vi "UNLOADING_CHECH_STATUS.vi"(0 "Unloading cyc Data":T1) -> (4 "DOOR NO.":string, 6 "QR Code":string, 8 "Unloading cyc Data OUT":T1)   [LabVIEW 2017]
uses:
  Controls/Feed_Cyc_Data.ctl
  Controls/Unloading_Cyc_Data.ctl
  <vilib>/Utility/file.llb/Read Delimited Spreadsheet (string).vi
  <vilib>/Utility/file.llb/Write Delimited Spreadsheet (string).vi
panel:
  in  "error in":errorcluster
  out "error out":errorcluster
  out "?":T2
  in  "Enum":enum16{"FEED", "LOADED"}(ring)=enum."LOADED"
  in  "Door No":i32
  out "output array":string[][](array[string])
  out "error out":errorcluster
  in  "error in (no error)":errorcluster
  in  "?":T2
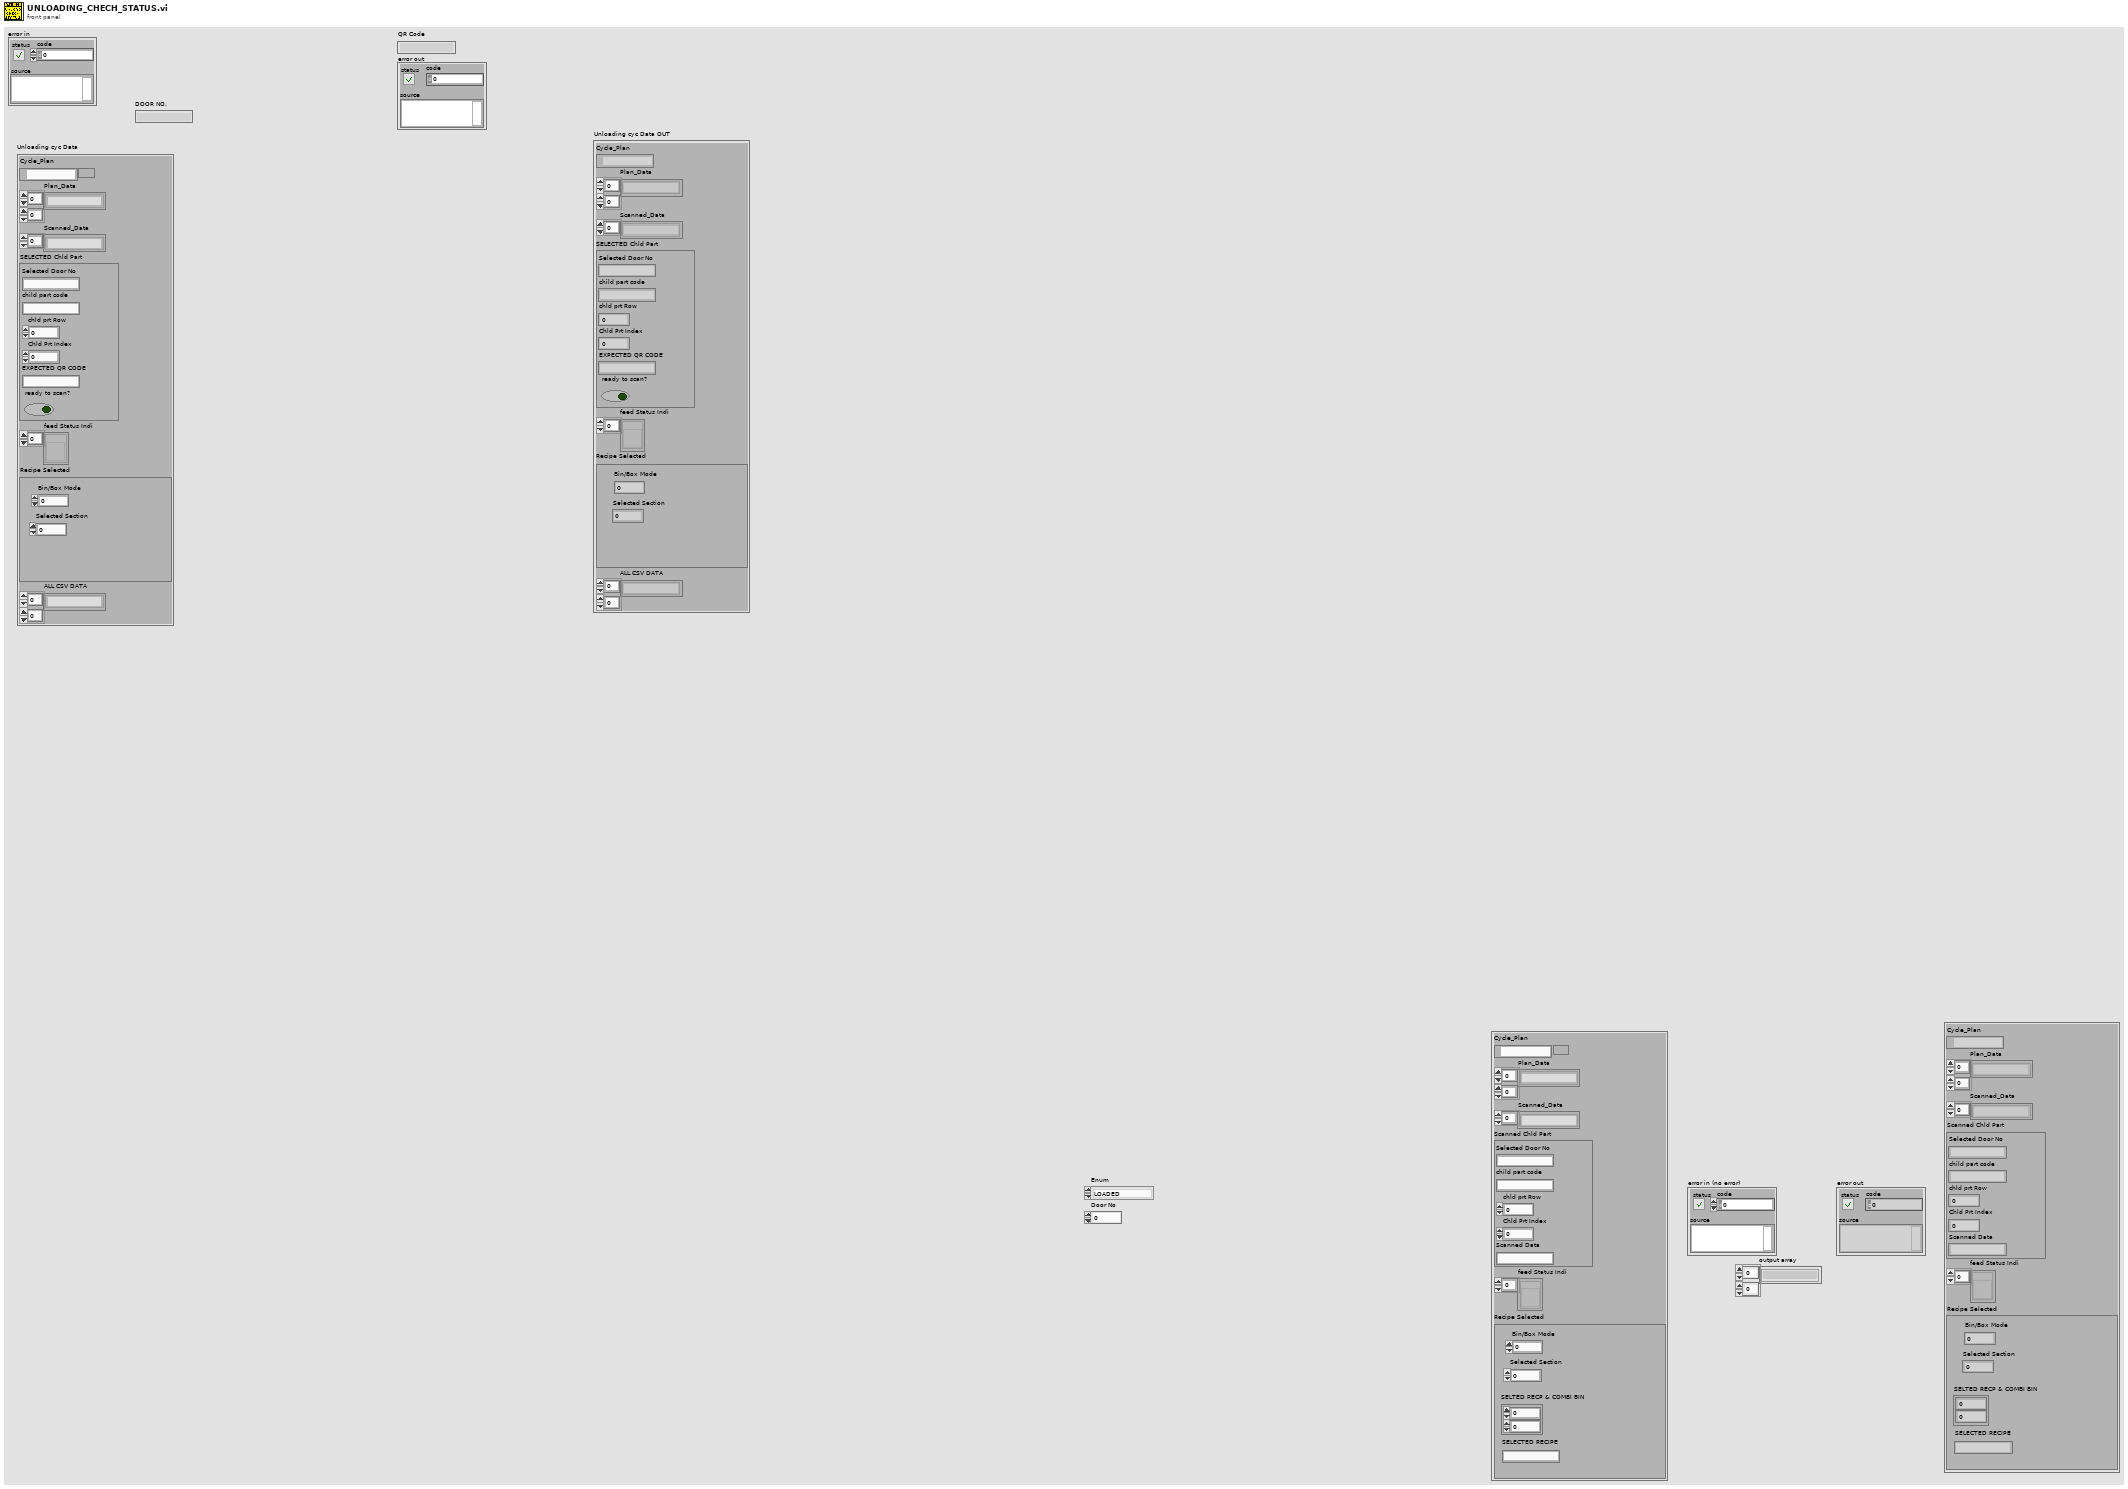
[diagram p1: front panel]
types:
  T1 = typedef "Unloading_Cyc_Data.ctl" = cluster{"Cycle_Plan":path, "Plan_Data":string[][], "Scanned_Data":string[], "SELECTED Chld Part":cluster{"Selected Door No":string, "child part code":string, "chld prt Row":i32, "Chld Prt Index":i32, "EXPECTED QR CODE":string, "ready to scan?":bool}, "feed Status Indi":refnum<vi>[], "Recipe Selected":cluster{"Bin/Box Mode":i32, "Selected Section":i32}, "ALL CSV DATA":string[][]}
  T2 = typedef "Feed_Cyc_Data.ctl" = cluster{"Cycle_Plan":path, "Plan_Data":string[][], "Scanned_Data":string[], "Scanned Chld Part":cluster{"Selected Door No":string, "child part code":string, "chld prt Row":i32, "Chld Prt Index":i32, "Scanned Data":string}, "feed Status Indi":refnum<vi>[], "Recipe Selected":cluster{"Bin/Box Mode":i32, "Selected Section":i32, "SELTED RECP & COMBI BIN":cluster{i32, i32}, "SELECTED RECIPE":string}}
  T3 = cluster{"Selected Door No":string, "child part code":string, "chld prt Row":i32, "Chld Prt Index":i32, "Scanned Data":string}
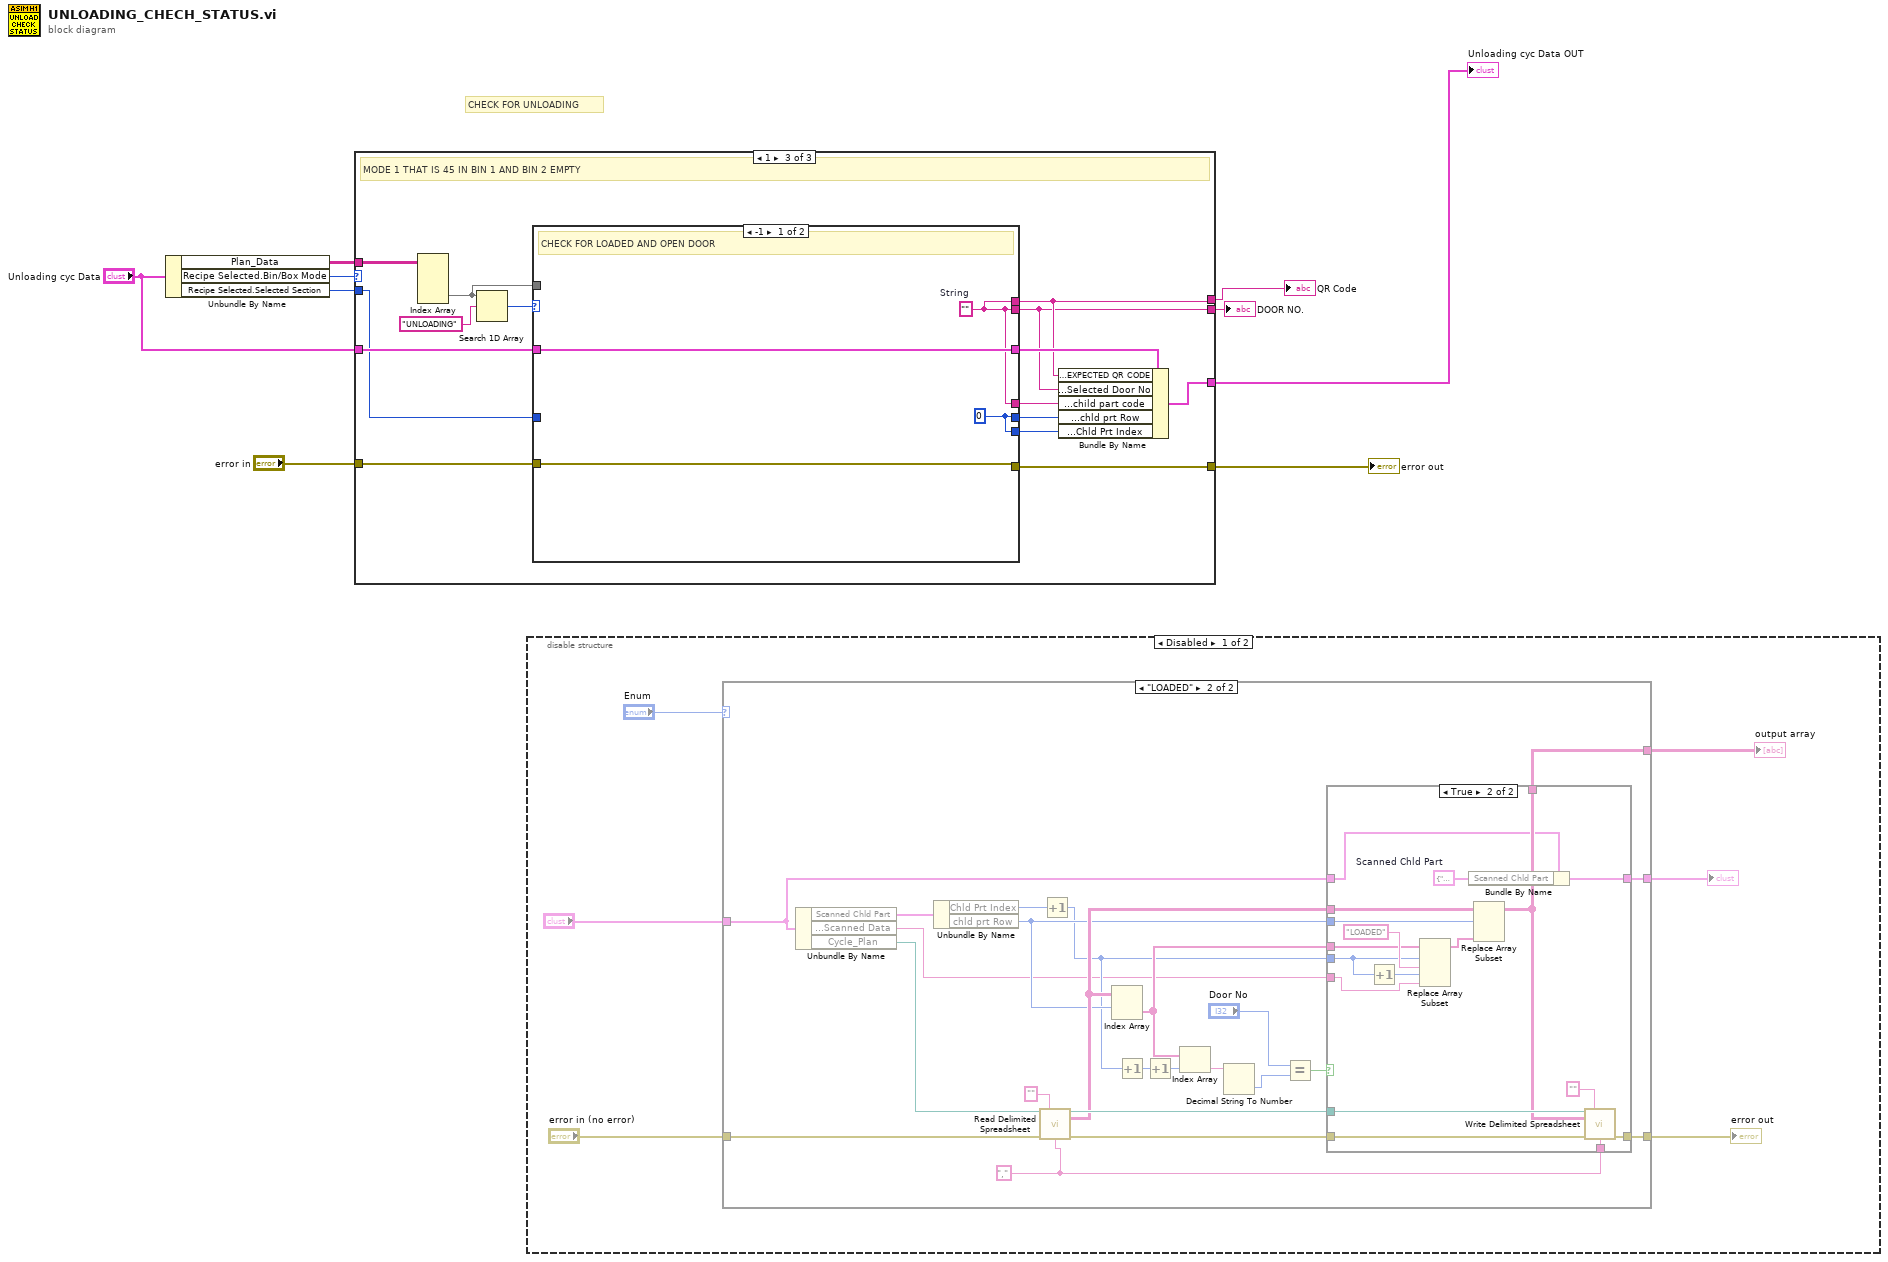
[diagram p0: block diagram]
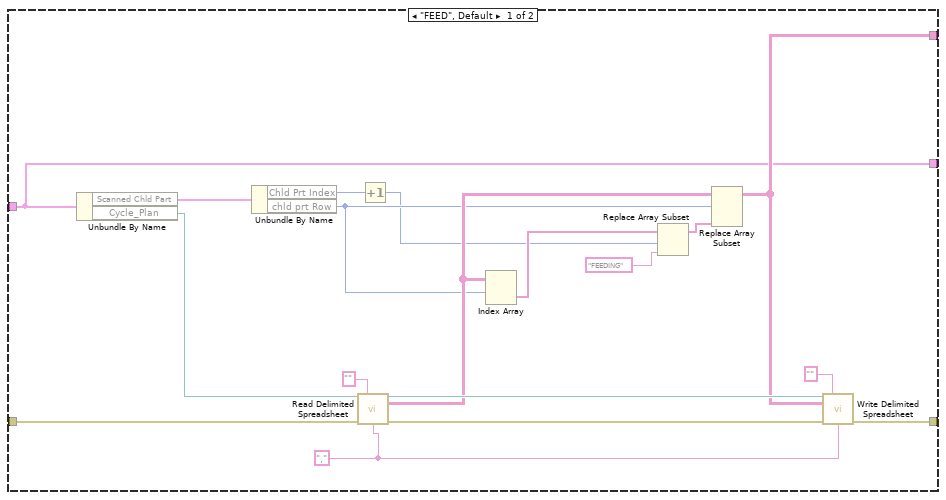
[diagram p2: hidden frame]
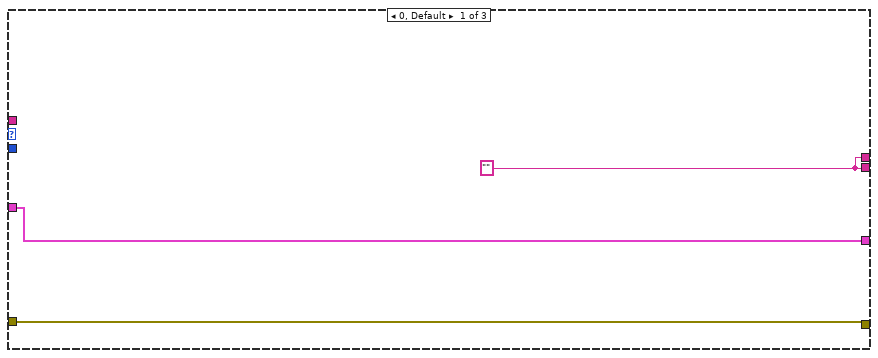
[diagram p5: hidden frame]
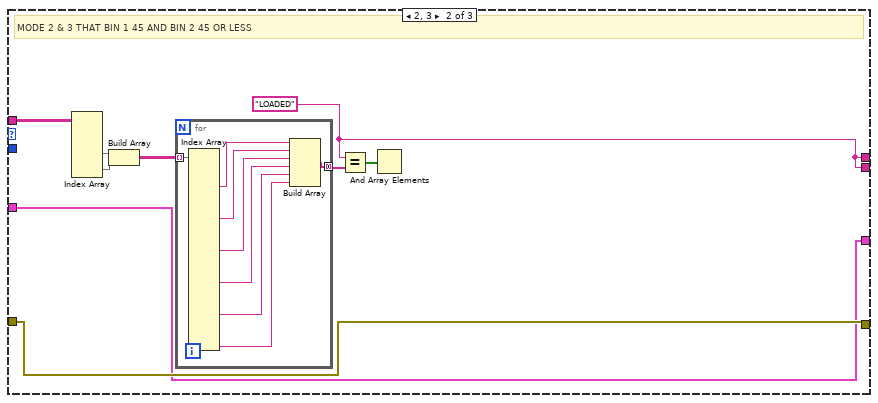
[diagram p6: hidden frame]
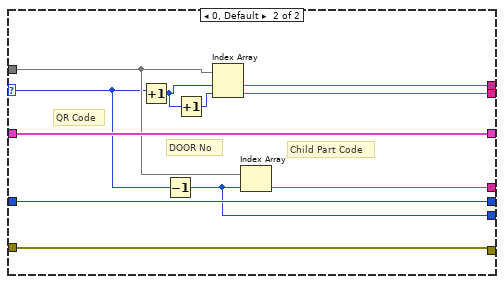
[diagram p7: hidden frame]
diagram:
  # "CHECK FOR UNLOADING"
  n1 = Unbundle By Name("Unloading cyc Data") -> ("Plan_Data"=w8:string[][], "Recipe Selected.Bin/Box Mode"=w7:i32, "Recipe Selected.Selected Section"=w5:i32)
  n2 = case shown="1" w7 {
    tunnel: w8 -> [_ w21 w44]
    tunnel: [w12 w15 w35] -> w9
    tunnel: [w12 w15 w36] -> w6
    tunnel: w5 -> [_ _ w31]
    tunnel: "Unloading cyc Data" -> [w10 w13 w43]
    tunnel: "error in" -> [w11 w14 w42]
    tunnel: [w11 w14 w41] -> w3
    tunnel: [w10 w13 w34] -> w1
    frame 0, Default {
      w12 = ""
    }
    frame 2, 3 {
      w15 = "LOADED"
      # "MODE 2 & 3 THAT BIN 1 45 AND BIN 2 45 OR LESS"
      n3 = Index Array(array=w21) -> (element #2=w20:string[], element #3=w19:string[])  [unwired: 6 in, 1 out]
      n4 = Build Array(w20, w19) -> (w18:string[][])
      n5 = for {
        tunnel: w18 -> [w29] mode=indexing
        tunnel: [w22] -> w17 mode=concatenating
        n6 = Index Array(array=w29) -> (element #3=w28:string, element #7=w27:string, element #11=w26:string, element #15=w25:string, element #19=w24:string, element #23=w23:string)  [unwired: 23 in, 17 out]
        n7 = Build Array(w28, w27, w26, w25, w24, w23) -> (w22:string[])
      }
      n8 = Equal?(x=w15, y=w17) -> (x = y?=w16:bool[])
      n9 = And Array Elements(Boolean array=w16) -> ()  [unwired: 1 out]
    }
    frame 1 {
      # "MODE 1 THAT IS 45 IN BIN 1 AND BIN 2 EMPTY"
      n10 = Index Array(array=w44) -> (element #2=w40:string[])  [unwired: 4 in, 1 out]
      n11 = Search 1D Array(1D array=w40, element="UNLOADING") -> (index of element=w38:i32)  [unwired: 1 in]
      n12 = case shown="-1" w38 {
        selector: w38 -> [_ w52]
        tunnel: [w46 w57] -> w35
        tunnel: w40 -> [_ w53]
        tunnel: [w46 w56] -> w36
        tunnel: w43 -> [w47 w54]
        tunnel: w42 -> [w48 w55]
        tunnel: [w48 w55] -> w41
        tunnel: [w47 w54] -> w37
        tunnel: [w46 w51] -> w33
        tunnel: [w45 w50] -> w32
        tunnel: w31 -> [_ w50]
        tunnel: [w45 w49] -> w30
        frame -1 {
          w45 = 0
          w46 = ""  # String
          # "CHECK FOR LOADED AND OPEN DOOR"
        }
        frame 0, Default {
          # "Child Part Code"
          # "QR Code"
          # "DOOR No"
          n13 = Increment(x=w52) -> (x+1=w58:i32)
          n14 = Decrement(x=w52) -> (x-1=w49:i32)
          n15 = Increment(x=w58) -> (x+1=w59:i32)
          n16 = Index Array(array=w53, index #1=w58, index #2=w59) -> (element #1=w56:string, element #2=w57:string)
          n17 = Index Array(array=w53, index=w49) -> (element=w51:string)
        }
      }
      n18 = Bundle By Name(cluster=w37, "SELECTED Chld Part.EXPECTED QR CODE"=w36, "SELECTED Chld Part.Selected Door No"=w35, "SELECTED Chld Part.child part code"=w33, "SELECTED Chld Part.chld prt Row"=w32, "SELECTED Chld Part.Chld Prt Index"=w30) -> (w34:T1)
    }
  }
  "DOOR NO." <- w9
  "QR Code" <- w6
  "error out" <- w3
  "Unloading cyc Data OUT" <- w1
  n19 = disable-structure shown="Disabled" {
    frame Disabled {
      n20 = case shown="\"LOADED\"" "Enum" {
        tunnel: "?" -> [w66 w87]
        tunnel: "error in (no error)" -> [w80 w104]
        tunnel: [w79 w103] -> w63
        tunnel: [w70 w99] -> w62
        tunnel: [w66 w86] -> w60
        frame "FEED", Default {
          w69 = ","
          n21 = Unbundle By Name(w66) -> ("Scanned Chld Part"=w78:T3, "Cycle_Plan"=w82:path)
          n22 = Unbundle By Name(w78) -> ("Chld Prt Index"=w74:i32, "chld prt Row"=w76:i32)
          n23 = call-poly <vilib>:"Read Delimited Spreadsheet.vi"("file path (dialog if empty)"=w82, "format (%s)"="", "error in (no error)"=w80, "delimiter (\\t)"=w69) -> ("new file path (Not A Path if cancelled)"=w81:path, "all rows"=w77:string[][], "error out"=w83:errorcluster)  [unwired: 6 in, 3 out]
          n24 = Increment(x=w74) -> (x+1=w73:i32)
          n25 = Index Array(array=w77, index (row)=w76) -> (element=w75:string[])  [unwired: 1 in]
          n26 = Replace Array Subset(array=w75, new element="FEEDING", index=w73) -> (w71:string[])
          n27 = Replace Array Subset(array=w77, new element=w71, index (row)=w76) -> (w70:string[][])  [unwired: 1 in]
          n28 = call-poly <vilib>:"Write Delimited Spreadsheet.vi"("file path (dialog if empty)"=w81, "format (%s)"="", "2D data"=w70, "error in (no error)"=w83, "delimiter (\\t)"=w69) -> ("error out"=w79:errorcluster)  [unwired: 9 in, 1 out]
        }
        frame "LOADED" {
          w98 = ","
          n29 = Unbundle By Name(w87) -> ("Scanned Chld Part"=w102:T3, "Scanned Chld Part.Scanned Data"=w85:string, "Cycle_Plan"=w84:path)
          n30 = Unbundle By Name(w102) -> ("Chld Prt Index"=w100:i32, "chld prt Row"=w96:i32)
          n31 = call-poly <vilib>:"Read Delimited Spreadsheet.vi"("file path (dialog if empty)"=w84, "format (%s)"="", "error in (no error)"=w104, "delimiter (\\t)"=w98) -> ("new file path (Not A Path if cancelled)"=w105:path, "all rows"=w101:string[][], "error out"=w106:errorcluster)  [unwired: 6 in, 3 out]
          n32 = Increment(x=w100) -> (x+1=w94:i32)
          n33 = Index Array(array=w101, index (row)=w96) -> (element=w95:string[])  [unwired: 1 in]
          n34 = Increment(x=w94) -> (x+1=w92:i32)
          n35 = Increment(x=w92) -> (x+1=w93:i32)
          n36 = Index Array(array=w95, index=w93) -> (element=w91:string)
          n37 = Decimal String To Number(string=w91) -> (number=w90:i32)  [unwired: 2 in, 1 out]
          n38 = Equal?(x="Door No", y=w90) -> (x = y?=w88:bool)
          n39 = case shown="True" w88 {
            tunnel: w106 -> [w108 w126]
            tunnel: w105 -> [_ w125]
            tunnel: [w108 w124] -> w103
            tunnel: w101 -> [w109 w123]
            tunnel: [w109 w120] -> w99
            tunnel: w98 -> [_ w119]
            tunnel: w96 -> [_ w118]
            tunnel: w95 -> [_ w117]
            tunnel: w94 -> [_ w111]
            tunnel: w87 -> [w107 w115]
            tunnel: [w107 w114] -> w86
            tunnel: w85 -> [_ w110]
            frame False {
            }
            frame True {
              w113 = T3 {"Selected Door No"="", "child part code"="", "chld prt Row"=0, "Chld Prt Index"=0, "Scanned Data"=""}  # Scanned Chld Part
              n40 = Increment(x=w111) -> (x+1=w112:i32)
              n41 = Replace Array Subset(array=w117, new element #1="LOADED", index #1=w111, new element #2=w110, index #2=w112) -> (w121:string[])
              n42 = Bundle By Name(cluster=w115, "Scanned Chld Part"=w113) -> (w114:T2)
              n43 = Replace Array Subset(array=w123, new element=w121, index (row)=w118) -> (w120:string[][])  [unwired: 1 in]
              n44 = call-poly <vilib>:"Write Delimited Spreadsheet.vi"("file path (dialog if empty)"=w125, "format (%s)"="", "2D data"=w120, "error in (no error)"=w126, "delimiter (\\t)"=w119) -> ("error out"=w124:errorcluster)  [unwired: 9 in, 1 out]
            }
          }
        }
      }
      "error out" <- w63
      "output array" <- w62
      "?" <- w60
    }
    frame Enabled {
    }
  }
